vi "TDMS_Close.vi"(8 "错误输入":errorcluster, 10 "队列Ref数组":refnum<queue>[](array[refnum]), 11 "tdms file":refnum<k34>) -> (0 "错误输出":errorcluster)   [LabVIEW 2011]
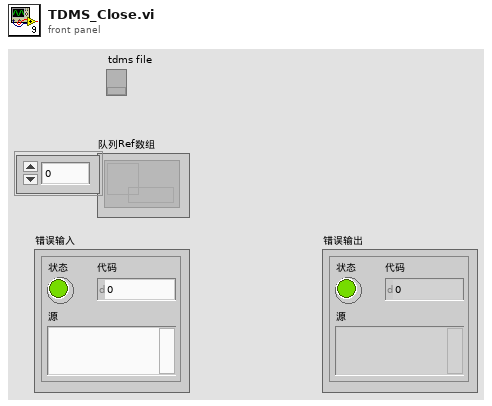
[diagram p1: front panel]
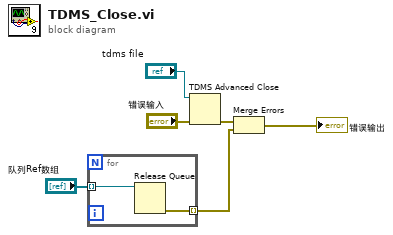
[diagram p0: block diagram]
diagram:
  n1 = for {
    tunnel: "队列Ref数组" -> [w8] mode=indexing
    tunnel: [w7] -> w3 mode=indexing
    n2 = Release Queue(queue=w8) -> (error out=w7:errorcluster)  [unwired: 2 in, 2 out]
  }
  n3 = TDMS Advanced Close(8:"错误输入", 11:"tdms file") -> (0:w4:errorcluster)  [unwired: 2 in, 1 out]
  n4 = Merge Errors(w4, w3) -> (→"错误输出":errorcluster)
